vi "Set Frequency.vi"(8 "error IO":errorcluster, 10 "Frequency":enum16{"50", "60", "400", "800"}(ring)=enum."60", 11 "VISA resource name":refnum<visa-resource-name>) -> (0 "error Out":errorcluster, 3 "VISA resource Out":refnum<visa-resource-name>)   [LabVIEW 2020, in "Associated Research 78XX Series.lvlib"]
uses:
  <instrlib>/Associated Research 78XX Series/Associated Research 78XX Series.lvlib
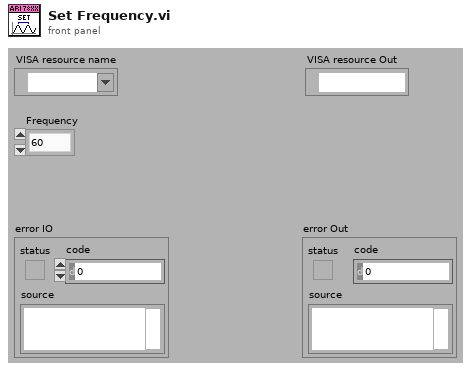
[diagram p1: front panel]
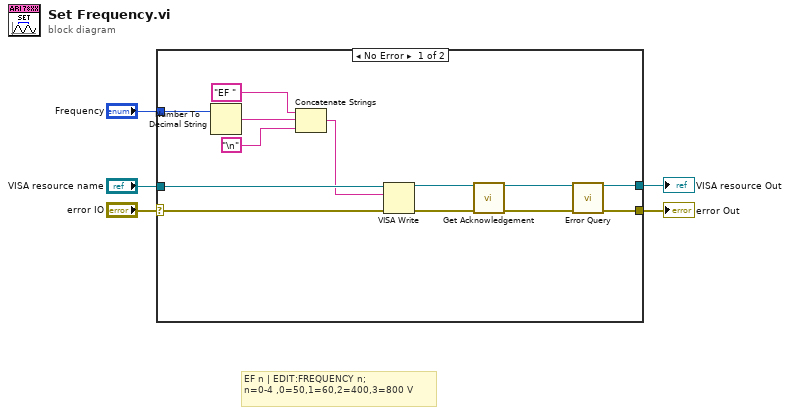
[diagram p0: block diagram]
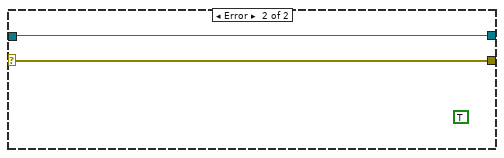
[diagram p2: hidden frame]
diagram:
  # "EF n\t| EDIT:FREQUENCY n;\nn=0-4 ,0=50,1=60,2=400,3=800\tV"
  n1 = case shown="No Error" "error IO" {
    selector: "error IO" -> [w18 w20]
    tunnel: [w15 w20] -> w2
    tunnel: [w16 w19] -> w3
    tunnel: "VISA resource name" -> [w17 w19]
    tunnel: "Frequency" -> [w14 _]
    frame No Error {
      n2 = Number To Decimal String(number=w14) -> (decimal integer string=w8:string)  [unwired: 1 in]
      n3 = Concatenate Strings("EF " ("Command to Send (empty)"), w8, "\n") -> (w11:string)
      n4 = VISA Write(VISA resource name=w17, write buffer=w11, error in (no error)=w18) -> (VISA resource name out=w7:refnum<visa-resource-name>, error out=w6:errorcluster)  [unwired: 1 out]
      n5 = call <instrlib>:"Get Acknowledgement.vi"("VISA resource name"=w7, "error in (no error)"=w6) -> ("VISA resource name out"=w10:refnum<visa-resource-name>, "error out"=w9:errorcluster)  [unwired: 12 in]
      n6 = call <instrlib>:"Error Query.vi"("VISA resource name"=w10, "error in (no error)"=w9) -> ("VISA resource name out"=w16:refnum<visa-resource-name>, "error out"=w15:errorcluster)  [unwired: 10 in, 2 out]
    }
    frame Error {
      (unwired) TRUE ("Command Acknowledged?")
    }
  }
  "VISA resource Out" <- w3
  "error Out" <- w2
